vi "System_Start Process Loops.vi"(8 "error in (no error)":errorcluster, 11 "System DVR":refnum<data-value>) -> (0 "error out":errorcluster, 3 "System DVR out":refnum<data-value>)   [LabVIEW 2015, in "System.lvclass"]
uses:
  System.lvclass
  System.lvclass/System.ctl
  Interface_Asset/Interface_Asset_Launch Process.vi
  Interface_Asset/Interface_Asset.lvclass
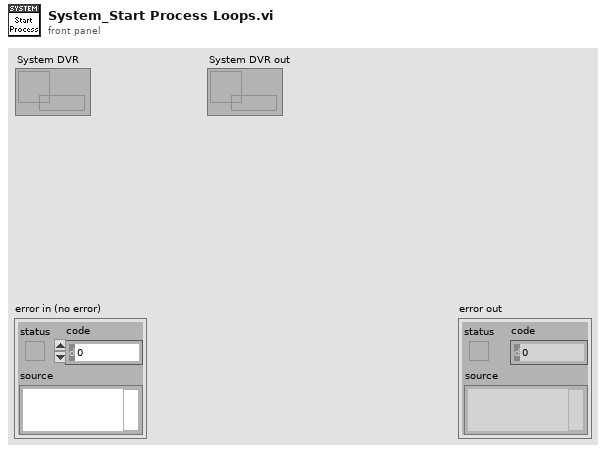
[diagram p1: front panel]
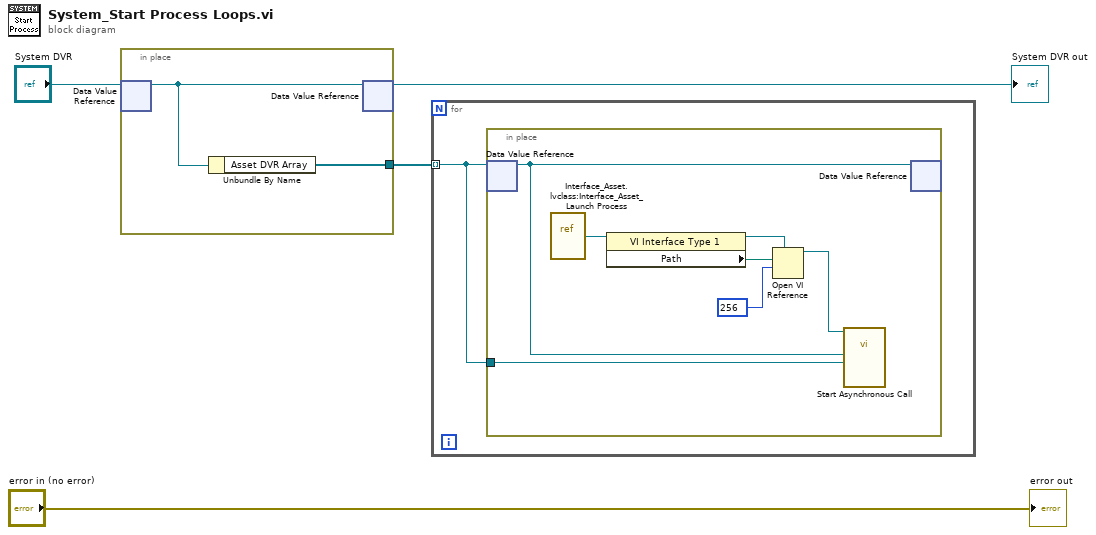
[diagram p0: block diagram]
diagram:
  n1 = in-place {
    in-place-border: [w5] -> w1
    n2 = in-place-dvr #1("System DVR") -> (w6:refnum<class "System.lvclass">)  [unwired: 1 out]
    n3 = Unbundle By Name(w6) -> ("Asset DVR Array"=w5:refnum<data-value>[])
    n4 = in-place-dvr #1(w6) -> (→"System DVR out":refnum<data-value>)  [unwired: 1 out]
  }
  n5 = for {
    tunnel: w1 -> [w7] mode=indexing
    n6 = in-place {
      in-place-border: w7 -> [w8]
      n7 = in-place-dvr #2(w7) -> (w9:refnum<class "Interface_Asset.lvclass">)  [unwired: 1 out]
      n8 = vi-ref "Interface_Asset.lvclass:Interface_Asset_Launch Process.vi"() -> (w14:refnum<vi>)
      n9 = property class="VI Interface Type 1"(reference=w14) -> (reference out=w12:refnum<vi>, "Path"=w11:path)  [unwired: 1 in, 1 out]
      n10 = Open VI Reference(type specifier VI Refnum (for type only)=w12, vi path=w11, options=256) -> (vi reference=w10:refnum<vi>)  [unwired: 3 in, 1 out]
      n11 = call-by-ref "Start Asynchronous Call"(reference=w10, "data value reference"=w8, "Interface_Asset in"=w9) -> ()  [unwired: 11 in, 2 out]
      n12 = in-place-dvr #2(w9) -> ()  [unwired: 2 out]
    }
  }
  "error out" <- "error in (no error)"
